vi "DetectFromVideo (1).vi"() -> ()   [LabVIEW 2021]
uses:
  <vilib>/vision/NI_Vision_Development_Module.lvlib
panel:
  out "Waveform Graph":sgl[](graph)
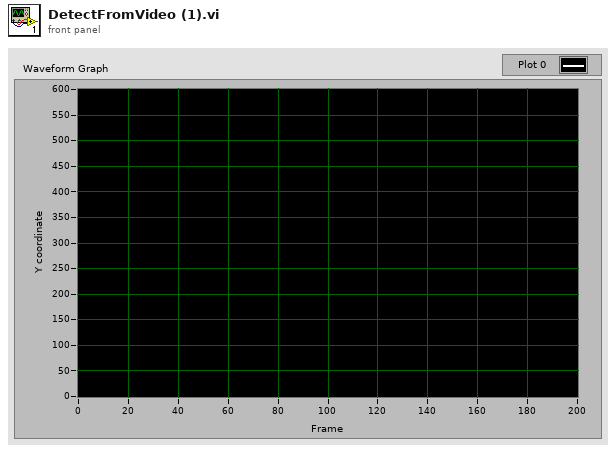
[diagram p1: front panel]
types:
  T1 = typedef "Image Type" = u32
  T2 = typedef "IMAQ Image.ctl" = refnum<image>
  T3 = typedef "IMAQ AVI2 Refnum.ctl" = refnum<k20>
  T4 = cluster{"Position":cluster{"x":sgl, "y":sgl}, "Angle":sgl, "Scale":sgl, "Score":sgl, "Bounding Box":cluster{"x":sgl, "y":sgl}[]}[]
  T5 = cluster{"Position":cluster{"x":sgl, "y":sgl}, "Angle":sgl, "Scale":sgl, "Score":sgl, "Bounding Box":cluster{"x":sgl, "y":sgl}[]}
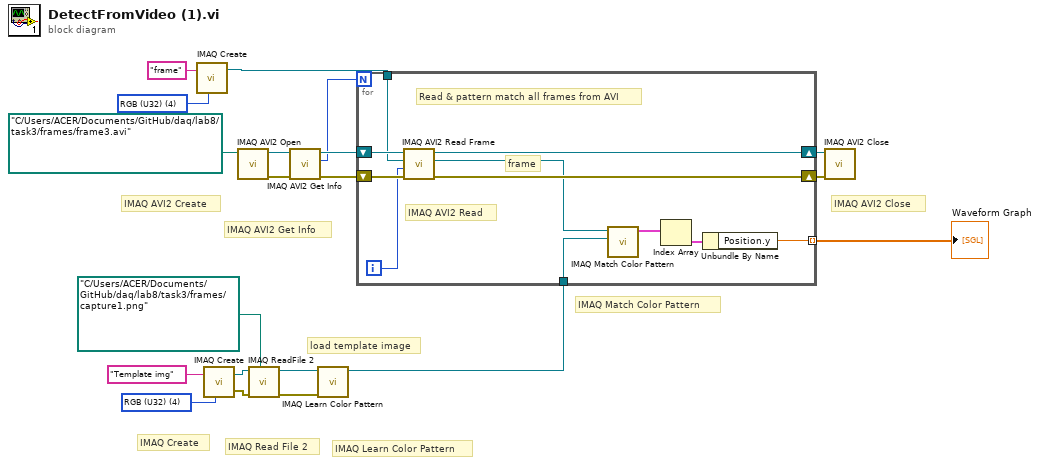
[diagram p0: block diagram]
diagram:
  w2 = T1 4 items=["Grayscale (U8)", "Grayscale (I16)", "Grayscale (SGL)", "Complex (CSG)", "RGB (U32)", "HSL (U32)", "RGB (U64)", "Grayscale (U16)"] ("Image Type")
  w16 = T1 4 items=["Grayscale (U8)", "Grayscale (I16)", "Grayscale (SGL)", "Complex (CSG)", "RGB (U32)", "HSL (U32)", "RGB (U64)", "Grayscale (U16)"] ("Image Type")
  # "load template image"
  # "IMAQ AVI2 Get Info"
  # "IMAQ Match Color Pattern"
  # "IMAQ Learn Color Pattern"
  # "IMAQ Create"
  # "IMAQ Read File 2"
  # "IMAQ AVI2 Close"
  # "IMAQ AVI2 Create"
  n1 = call "IMAQ Create"("Image Name"="frame", "Image Type"=w2) -> ("New Image"=w1:T2)  [unwired: 3 in, 1 out]
  n2 = call "IMAQ Create"("Image Name"="Template img", "Image Type"=w16) -> ("New Image"=w14:T2, "error out"=w12:errorcluster)  [unwired: 3 in]
  n3 = call "IMAQ AVI2 Open"("AVI File Path"=path "C:/Users/ACER/Documents/GitHub/daq/lab8/task3/frames/frame3.avi" ("AVI Path")) -> ("error out"=w6:errorcluster, "AVI Refnum"=w7:T3)  [unwired: 9 in]
  n4 = call "IMAQ ReadFile 2"("File Path"=path "C:/Users/ACER/Documents/GitHub/daq/lab8/task3/frames/capture1.png", "error in (no error)"=w12, "Image"=w14) -> ("error out"=w11:errorcluster, "Image Out"=w10:T2)  [unwired: 4 in, 3 out]
  n5 = call "IMAQ AVI2 Get Info"("error in (no error)"=w6, "AVI Refnum"=w7) -> ("error out"=w5:errorcluster, "Number of Frames"=w3:u32, "AVI Refnum (duplicate)"=w4:T3)  [unwired: 5 in, 2 out]
  n6 = call "IMAQ Learn Color Pattern"("error in (no error)"=w11, "Image"=w10) -> ("Template Image Out"=w9:T2)  [unwired: 8 in, 1 out]
  n7 = for {
    N: w3 -> [_]
    shift-right: [w29] -> w19
    shift-left: w4 -> [w30]
    shift-right: [w28] -> w20
    shift-left: w5 -> [w31]
    tunnel: w9 -> [w27]
    tunnel: [w25] -> w8 mode=indexing
    tunnel: w1 -> [w22]
    i -> [w23]
    # "Read & pattern match all frames from AVI"
    # "IMAQ AVI2 Read"
    # "frame"
    n8 = call "IMAQ AVI2 Read Frame"("error in (no error)"=w31, "Frame Number"=w23, "Image"=w22, "AVI Refnum"=w30) -> ("error out"=w28:errorcluster, "Image Out"=w24:T2, "AVI Refnum (duplicate)"=w29:T3)  [unwired: 5 in]
    n9 = call "IMAQ Match Color Pattern"("Template Image"=w27, "Image"=w24) -> ("Matches"=w26:T4)  [unwired: 7 in, 2 out]
    n10 = Index Array "Index Array"(array=w26) -> (element=w21:T5)  [unwired: 1 in]
    n11 = Unbundle By Name "Unbundle By Name"(w21) -> ("Position.y"=w25:sgl)
  }
  "Waveform Graph" <- w8
  n12 = call "IMAQ AVI2 Close"("error in (no error)"=w20, "AVI Refnum"=w19) -> ()  [unwired: 9 in, 1 out]
